vi "PQoidStatus.vi"(8 "error in (no error)":errorcluster, 11 "res":u64) -> (0 "error out":errorcluster, 3 "PQoidStatus":string)   [LabVIEW 2019, in "libpqlv64.lvlib"]
uses:
  libpqlv64.lvlib
  libpq.dll
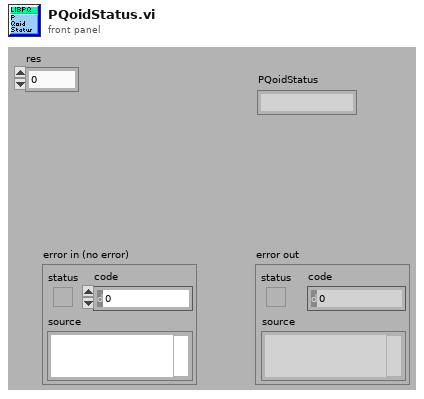
[diagram p1: front panel]
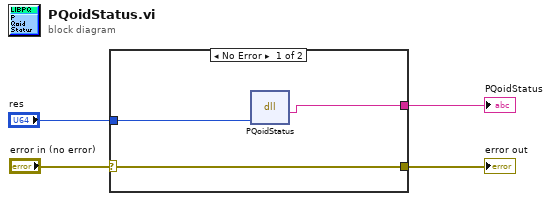
[diagram p0: block diagram]
diagram:
  n1 = case shown="No Error" "error in (no error)" {
    selector: "error in (no error)" -> [w7 w8]
    tunnel: [w7 w8] -> w3
    tunnel: [w6 _] -> w2
    tunnel: "res" -> [w5 _]
    frame No Error {
      n2 = dll-call lib="libpq.*" fn="PQoidStatus"("res"=w5) -> ("PQoidStatus"=w6:string)  [unwired: 4 in, 2 out]
    }
    frame Error {
    }
  }
  "PQoidStatus" <- w2
  "error out" <- w3
